vi "Run all tests.vi"(8 "error in (no error)":errorcluster, 10 "Interactive (T)":bool=TRUE, 11 "Test Report":refnum<class "Test Report.lvclass">) -> (0 "error out":errorcluster, 2 "Report":path, 3 "Test Results":refnum<class "Test Result.lvclass">)   [LabVIEW 2021]
uses:
  <vilib>/addons/_JKI Toolkits/Caraya/classes/Test Result/Test Result.lvclass
  <vilib>/addons/_JKI Toolkits/Caraya/classes/Test Report/Test Report.lvclass
  <vilib>/addons/_JKI Toolkits/Caraya/run-tests/Run Test (Scalar Path).vi
  <vilib>/addons/_JKI Toolkits/Caraya/Caraya.lvlib
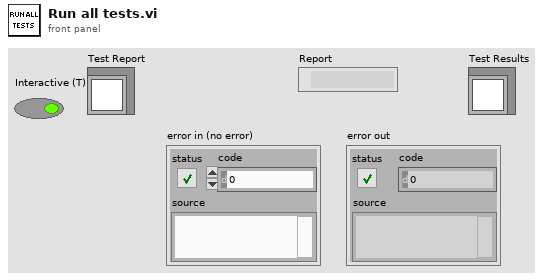
[diagram p1: front panel]
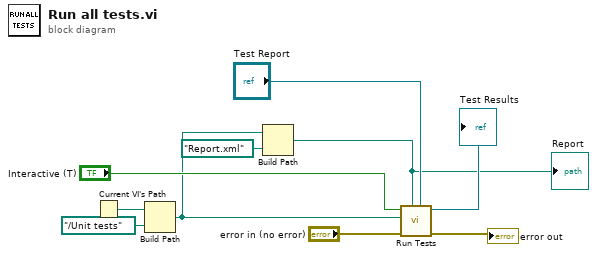
[diagram p0: block diagram]
diagram:
  n1 = Current VI's Path() -> (path=w10:path)
  n2 = Build Path(base path=w10, name or relative path=path "../Unit tests") -> (appended path=w5:path)
  n3 = Build Path(base path=w5, name or relative path=path "Report.xml") -> (appended path=w3:path)
  "Report" <- w3
  n4 = call-poly <vilib>:"Run Tests.vi"("Test Report"="Test Report", "Report Path"=w3, "error in"="error in (no error)", "Test Path"=w5, "Interactive (T)"="Interactive (T)") -> ("error out"=→"error out":errorcluster, "Test Results"=→"Test Results":refnum<class "Test Result.lvclass">)  [unwired: 5 in]
